vi "Seperate Signal Name and Parameters.vi"(11 "String":string) -> (2 "Signal Parameters":string[](array[string]), 3 "Signal Name":string)   [LabVIEW 2019, in "Diagnostics Addon System Explorer.lvlib"]
uses:
  Diagnostics Addon System Explorer.lvlib
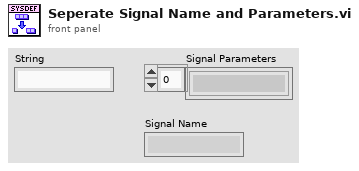
[diagram p1: front panel]
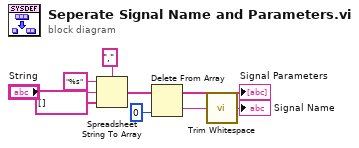
[diagram p0: block diagram]
diagram:
  n1 = Spreadsheet String To Array(delimiter (Tab)=",", format string="%s", spreadsheet string="String", array type (2D Dbl)=string[] []) -> (array=w5:string[])
  n2 = Delete From Array(array=w5, index=0) -> (deleted portion=w8:string, array with subset deleted=→"Signal Parameters":string[])  [unwired: 1 in]
  n3 = call <vilib>:"Trim Whitespace.vi"("string"=w8) -> ("trimmed string"=→"Signal Name":string)  [unwired: 1 in]
